vi "CPU_clock_ticks_lookup.vi"(11 "opcode":u8 format="%02x") -> (3 "clock ticks":u32)   [LabVIEW 2018]
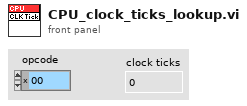
[diagram p1: front panel]
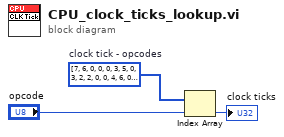
[diagram p0: block diagram]
diagram:
  w1 = u32[] [7, 6, 0, 0, 0, 3, 5, 0, 3, 2, 2, 0, 0, 4, 6, 0, 2, 5, 0, 0, 0, 4, 6, 0, 2, 4, 0, 0, 0, 4, 7, 0, 6, 6, 0, 0, 3, 3, 5, 0, 4, 2, 2, 0, 4, 4, 6, 0, 2, 5, 0, 0, 0, 4, 6, 0, 2, 4, 0, 0, 0, 4, 7, 0, 6, 6, 0, 0, 0, 3, 5, 0, 3, 2, 2, 0, 3, 4, 6, 0, 2, 5, 0, 0, 0, 4, 6, 0, 2, 4, 0, 0, 0, 4, 7, 0, 6, 6, 0, 0, 0, 3, 5, 0, 4, 2, 2, 0, 5, 4, 6, 0, 2, 5, 0, 0, 0, 4, 6, 0, 2, 4, 0, 0, 0, 4, 7, 0, 0, 6, 0, 0, 3, 3, 3, 0, 2, 0, 2, 0, 4, 4, 4, 0, 2, 6, 0, 0, 4, 4, 4, 0, 2, 5, 2, 0, 0, 5, 0, 0, 2, 6, 2, 0, 3, 3, 3, 0, 2, 2, 2, 0, 4, 4, 4, 0, 2, 5, 0, 0, 4, 4, 4, 0, 2, 4, 2, 0, 4, 4, 4, 0, 2, 6, 0, 0, 3, 3, 5, 0, 2, 2, 2, 0, 4, 4, 6, 0, 2, 5, 0, 0, 0, 4, 6, 0, 2, 4, 0, 0, 0, 4, 7, 0, 2, 6, 0, 0, 3, 3, 5, 0, 2, 2, 2, 0, 4, 4, 6, 0, 2, 5, 0, 0, 0, 4, 6, 0, 2, 4, 0, 0, 0, 4, 7, 0]  # clock tick - opcodes
  n1 = Index Array(array=w1, index="opcode") -> (element=→"clock ticks":u32)
